vi "Coord list setup unbundler-DBL.vi"(8 "error in (no error)":errorcluster, 9 "Keys Array":T1, 10 "Section":string, 11 "User profile ref":T2) -> (0 "error out":errorcluster, 3 "User profile ref":T2)   [LabVIEW 2020]
uses:
  <vilib>/Utility/config.llb/Config Data RefNum.ctl
  Typedefs/Ini file interface (DBL).ctl
  User Interface/Windows/Coordinates list window/Globals/Coord window-Globals.vi
  <vilib>/Utility/config.llb/NI_LVConfig.lvlib
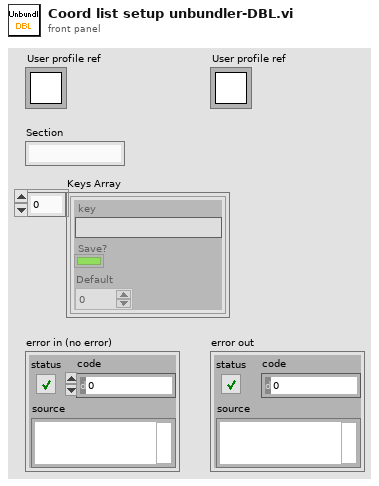
[diagram p1: front panel]
types:
  T1 = typedef "Ini file interface (DBL).ctl" = cluster{"key":string, "Save?":bool, "Default":dbl}[]
  T2 = typedef "NI_LVConfig.lvlib/Config Data RefNum.ctl" = refnum<k1>
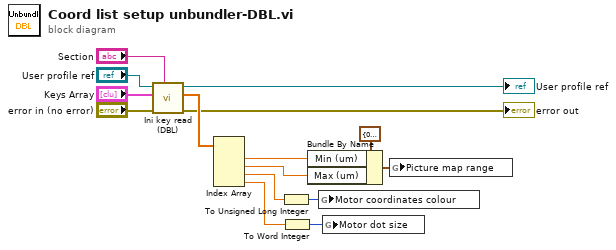
[diagram p0: block diagram]
diagram:
  n1 = call "Ini key read (DBL).vi"("Section name"="Section", "error in (no error)"="error in (no error)", "Parameter names & setup"="Keys Array", "Ini file refnum in"="User profile ref") -> ("error out"=→"error out":errorcluster, "Value read/used"=w7:dbl[], "Ini file refnum out"=→"User profile ref":T2)  [unwired: 5 in]
  n2 = Index Array(array=w7) -> (element #1=w6:dbl, element #2=w5:dbl, element #3=w4:dbl, element #4=w3:dbl)  [unwired: 4 in]
  n3 = To Unsigned Long Integer(number=w4) -> (unsigned 32bit integer=w14:u32)
  n4 = To Word Integer(number=w3) -> (16bit integer=w15:i16)
  n5 = Bundle By Name(cluster=cluster{"Min (um)":dbl, "Max (um)":dbl} {"Min (um)"=0.0, "Max (um)"=0.0} ("Picture map range"), "Min (um)"=w6, "Max (um)"=w5) -> (w13:cluster{"Min (um)":dbl, "Max (um)":dbl})
  n6 = global write "Coord window-Globals.vi" "Motor coordinates colour"(w14) -> ()
  n7 = global write "Coord window-Globals.vi" "Motor dot size"(w15) -> ()
  n8 = global write "Coord window-Globals.vi" "Picture map range"(w13) -> ()
